vi "2D Guassian - Fit Image DBL.vi"(7 "Image In (DBL)":dbl[][](array[numeric])) -> (8 "Best Fit Params":T1)   [LabVIEW 2016]
uses:
  2D Gaussian - Type Defs/2D Gaussian - Best Fit Parameters.ctl
  <vilib>/gmath/NumericalOptimization/Nonlinear Curve Fit LM bound.vi
  <vilib>/gmath/NI_Gmath.lvlib
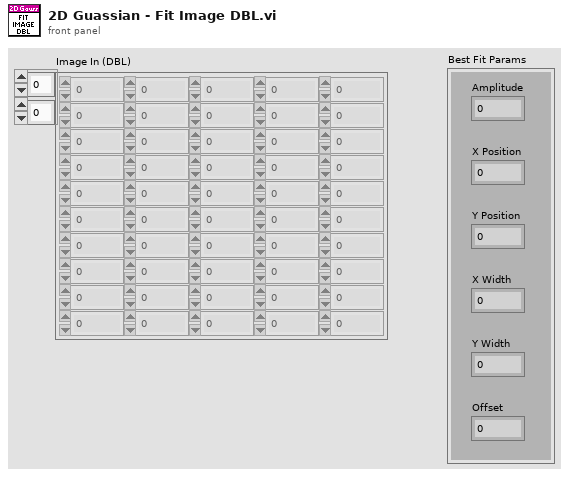
[diagram p1: front panel]
types:
  T1 = typedef "2D Gaussian - Best Fit Parameters.ctl" = cluster{"Amplitude":dbl, "X Position":dbl, "Y Position":dbl, "X Width":dbl, "Y Width":dbl, "Offset":dbl}
  T2 = cluster{"parameter minimum":dbl[], "parameter maximum":dbl[]}
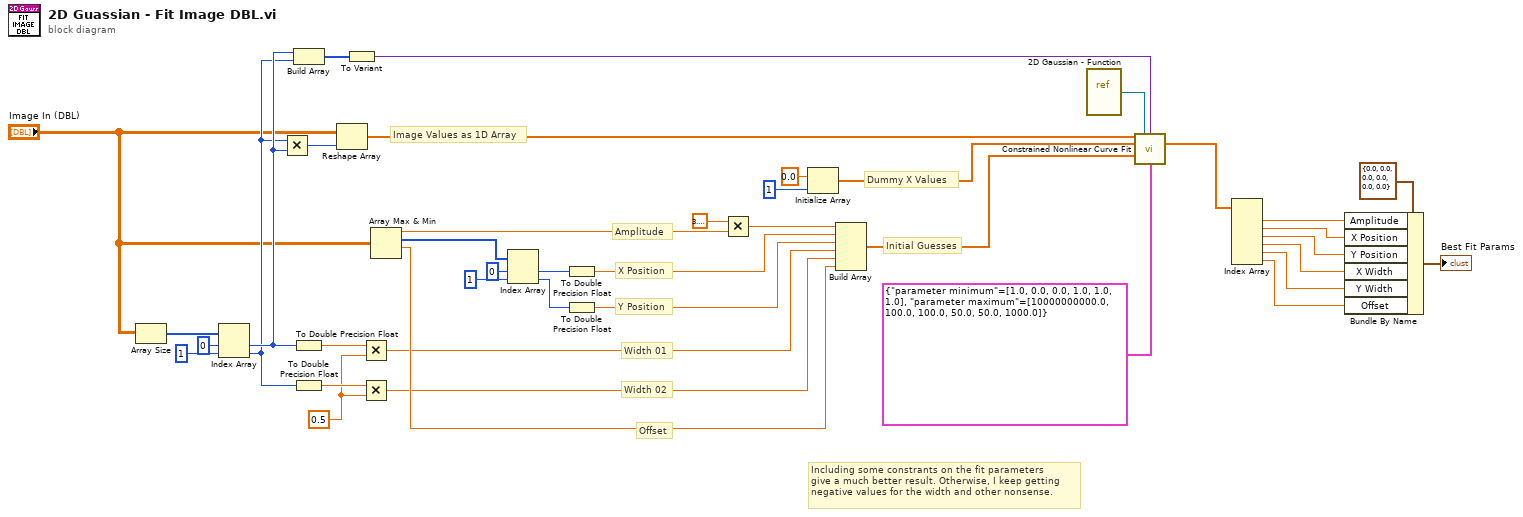
[diagram p0: block diagram]
diagram:
  w24 = 0.5
  # "Including some constrants on the fit parameters\ngive a much better result. Otherwise, I keep getting\nnegative values for the width and other nonsense."
  # "Dummy X Values"
  # "Image Values as 1D Array"
  # "Initial Guesses"
  # "Width 02"
  # "Width 01"
  # "Y Position"
  # "X Position"
  # "Offset"
  # "Amplitude"
  n1 = Array Size(array="Image In (DBL)") -> (size(s)=w27:i32[])
  n2 = Index Array(array=w27, index #1=0 ("index"), index #2=1 ("index")) -> (element #1=w15:i32, element #2=w14:i32)
  n3 = Multiply(x=w14, y=w15) -> (x*y=w20:i32)
  n4 = Build Array(w15, w14) -> (w13:i32[])
  n5 = To Double Precision Float(number=w15) -> (double precision float=w26:dbl)
  n6 = To Double Precision Float(number=w14) -> (double precision float=w25:dbl)
  n7 = Reshape Array("Image In (DBL)", w20) -> (w21:dbl[])
  n8 = To Variant(anything=w13) -> (Variant=w12:variant)
  n9 = Multiply(x=w26, y=w24) -> (x*y=w23:dbl)
  n10 = Multiply(x=w25, y=w24) -> (x*y=w22:dbl)
  n11 = Array Max & Min(array="Image In (DBL)") -> (max value=w39:dbl, max index (indices)=w36:i32[], min value=w37:dbl)  [unwired: 1 out]
  n12 = Index Array(array=w36, index #1=0 ("index"), index #2=1 ("index")) -> (element #1=w33:i32, element #2=w31:i32)
  n13 = To Double Precision Float(number=w33) -> (double precision float=w32:dbl)
  n14 = To Double Precision Float(number=w31) -> (double precision float=w30:dbl)
  n15 = Multiply(x=3.141592653589793, y=w39) -> (x*y=w38:dbl)
  n16 = Initialize Array(0.0 ("element"), 1 ("dimension size")) -> (w18:dbl[])
  n17 = Build Array(w38, w32, w30, w23, w22, w37) -> (w17:dbl[])
  n18 = vi-ref "2D Gaussian - Function.vi"() -> (w41:refnum<vi>)
  n19 = call-poly <vilib>:"Constrained Nonlinear Curve Fit.vi"("Y"=w21, "f(x,a)"=w41, "data"=w12, "X"=w18, "initial parameters"=w17, "parameter bounds"=T2 {"parameter minimum"=[1.0, 0.0, 0.0, 1.0, 1.0, 1.0], "parameter maximum"=[10000000000.0, 100.0, 100.0, 50.0, 50.0, 1000.0]}) -> ("best fit parameters"=w10:dbl[])  [unwired: 4 in, 5 out]
  n20 = Index Array(array=w10) -> (element #1=w9:dbl, element #2=w8:dbl, element #3=w7:dbl, element #4=w6:dbl, element #5=w5:dbl, element #6=w4:dbl)  [unwired: 6 in]
  n21 = Bundle By Name(cluster=T1 {"Amplitude"=0.0, "X Position"=0.0, "Y Position"=0.0, "X Width"=0.0, "Y Width"=0.0, "Offset"=0.0} ("Best Fit Parameters"), "Amplitude"=w9, "X Position"=w8, "Y Position"=w7, "X Width"=w6, "Y Width"=w5, "Offset"=w4) -> (→"Best Fit Params":T1)
